vi "Write Timeout.vi"(8 "error in":errorcluster, 10 "Timeout?":bool, 11 "Popup in":refnum<class "Popup.lvclass">) -> (0 "error out":errorcluster, 3 "Popup out":refnum<class "Popup.lvclass">)   [LabVIEW 2021, in "Pop-Up.lvlib" / "Popup.lvclass"]
doc: "This Data Member Access VI will write the timeout Boolean on the object.\n\nOutputs\n-Timeout [Boolean] - the result of the timeout\n\n<b>Code Developed By:</b>\nDaniel Coons\nTechnology Service Corporation\n1983 S Liberty Drive\nBloomington, IN 47403\nPhone: 812 558-7100\ndaniel.coons@tsc.com\nwww.tsc.com/atcs"
uses:
  Popup.lvclass
  Popup.lvclass/Popup.ctl
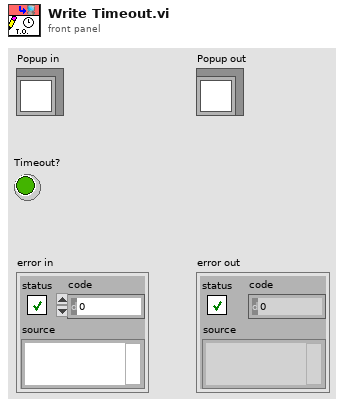
[diagram p1: front panel]
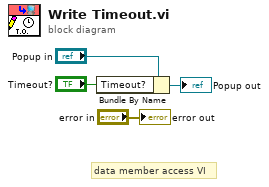
[diagram p0: block diagram]
diagram:
  # "data member access VI"
  n1 = Bundle By Name(cluster="Popup in", "Timeout?"="Timeout?") -> (→"Popup out":refnum<class "Popup.lvclass">)
  "error out" <- "error in"
